vi "writeTriggeringXML.vi"(8 "error in (no error)":errorcluster, 10 "NativeXML in":refnum<class "NativeXML.lvclass">, 11 "PixelflySettings in":refnum<class "PixelflySettings.lvclass">) -> (0 "error out":errorcluster, 2 "NativeXML out":refnum<class "NativeXML.lvclass">, 3 "PixelflySettings out":refnum<class "PixelflySettings.lvclass">)   [LabVIEW 2011, in "Tools.lvlib" / "Settings.lvlib" / "PixelflySettings.lvclass"]
uses:
  PixelflySettings.lvclass
  NativeXML/NativeXML.lvclass
  PixelflySettings.lvclass/PixelflySettings.ctl
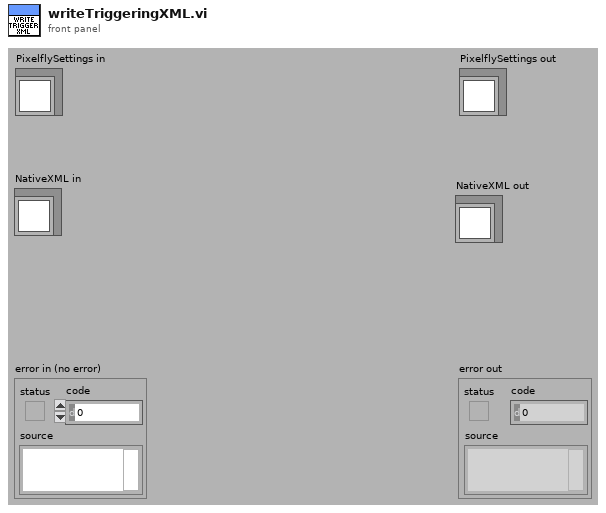
[diagram p1: front panel]
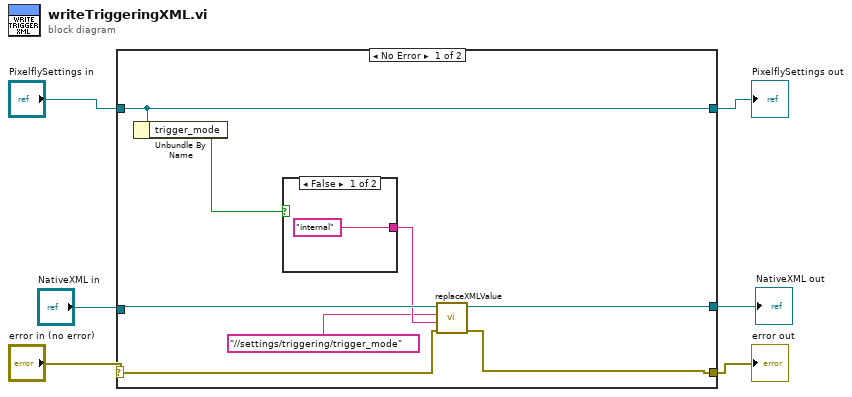
[diagram p0: block diagram]
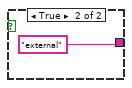
[diagram p2: hidden frame]
diagram:
  n1 = case shown="No Error" "error in (no error)" {
    selector: "error in (no error)" -> [w8 w19]
    tunnel: [w7 w19] -> w4
    tunnel: [w14 w18] -> w5
    tunnel: "PixelflySettings in" -> [w14 w18]
    tunnel: "NativeXML in" -> [w12 w17]
    tunnel: [w11 w17] -> w2
    frame No Error {
      n2 = Unbundle By Name(w14) -> ("trigger_mode"=w13:bool)
      n3 = case shown="False" w13 {
        tunnel: ["internal" "external"] -> w10
        frame False {
        }
        frame True {
        }
      }
      n4 = call "replaceXMLValue.vi"("error in (no error)"=w8, "value"=w10, "replace in"="//settings/triggering/trigger_mode", "NativeXML in"=w12) -> ("error out"=w7:errorcluster, "NativeXML out"=w11:refnum<class "NativeXML.lvclass">)  [unwired: 6 in]
    }
    frame Error {
    }
  }
  "error out" <- w4
  "PixelflySettings out" <- w5
  "NativeXML out" <- w2
